vi "Actor Core.vi"(8 "error in":errorcluster, 11 "UserInterface in":refnum<class "UserInterface.lvclass">) -> (0 "error out":errorcluster, 3 "Actor out":refnum<class "Actor.lvclass">)   [LabVIEW 2022 SP3, in "UserInterface.lvlib" / "UserInterface.lvclass"]
doc: "(<B>Filename</B>: Actor Framework.lvlib:Actor.lvclass:Actor Core.vi)\n\nReceives messages to the actor, reacts to them, and initiates any error handling that may shut the actor down.\n\nDescendant classes may override this VI to append parallel tasks for the actor to complete while it handles messages. Overrides use the Call Parent Class Method node."
uses:
  UserInterface.lvclass
  C:/Program Files/National Instruments/LabVIEW 2022/vi.lib/ActorFramework/Actor/Actor.lvclass
  <vilib>/ActorFramework/Actor/Actor.lvclass
  Typedefs/Image Formats.ctl
  Helper Loop Status.ctl
  UserInterface.lvclass/UserInterface.ctl
  <vilib>/ActorFramework/Actor/Actor.lvclass/Actor.ctl
  UI - Controller -- Interface Messages/Component Name Msg/Component Name Msg.lvclass/Component Name Msg.ctl
  <vilib>/ActorFramework/Message Enqueuer/Message Enqueuer.lvclass/Message Enqueuer.ctl
  UI - Controller -- Interface Messages/Total Images Msg/Total Images Msg.lvclass/Total Images Msg.ctl
  UI - Controller -- Interface Messages/Image Type Msg/Image Type Msg.lvclass/Image Type Msg.ctl
  UserInterface Messages/Total Images Msg/Total Images Msg.lvclass/Total Images Msg.ctl
  UI - Controller -- Interface Messages/Image Indicator Ref Msg/Image Indicator Ref Msg.lvclass/Image Indicator Ref Msg.ctl
  UI - Controller -- Interface Messages/Display Image Msg/Display Image Msg.lvclass/Display Image Msg.ctl
  <vilib>/ActorFramework/Message Enqueuer/Enqueue.vi
  <vilib>/ActorFramework/Message Enqueuer/Init from Existing Queue.vi
  UI - Controller -- Interface Messages/Component Name Msg/Component Name Msg.lvclass
  C:/Program Files/National Instruments/LabVIEW 2022/vi.lib/ActorFramework/Message/Message.lvclass
  UI - Controller -- Interface Messages/Total Images Msg/Total Images Msg.lvclass
  UI - Controller -- Interface Messages/Image Type Msg/Image Type Msg.lvclass
  UI - Controller -- Interface Messages/StartHarvest Msg/StartHarvest Msg.lvclass
  UI - Controller -- Interface Messages/StopHarvest Msg/StopHarvest Msg.lvclass
  UserInterface Messages/Total Images Msg/Total Images Msg.lvclass
  UI - Controller -- Interface Messages/Launch Calibration Msg/Launch Calibration Msg.lvclass
  UI - Controller -- Interface Messages/Image Request Msg/Image Request Msg.lvclass
  UI - Controller -- Interface Messages/Launch Settings Msg/Launch Settings Msg.lvclass
  UI - Controller -- Interface Messages/Open Folder Msg/Open Folder Msg.lvclass
  UI - Controller -- Interface Messages/Image Indicator Ref Msg/Image Indicator Ref Msg.lvclass
  UserInterface Messages/Reset UI Msg/Reset UI Msg.lvclass
  <vilib>/ActorFramework/Stop Msg/Stop Msg.lvclass
  UI - Controller -- Interface Messages/Display Image Msg/Display Image Msg.lvclass
  <vilib>/ActorFramework/Message Priority Queue/Priority Enqueue.vi
  <vilib>/ActorFramework/Message Enqueuer/Message Enqueuer.lvclass
  UserInterface.lvlib
panel:
  out "PLC":bool caption="PLC Not Ready"
  out "Image Sensor":bool caption="Sensor Not Ready"
  out "Version":string
  in  "Total Images":u32
  in  "Image Format":T1
  in  "Component Name":string
  in  "Open Folder":bool
  in  "Calibration":bool
  in  "Settings":bool
  in  "Stop":bool
  in  "Start":bool
  out "?":string
  in  "Trigger":bool
  in  "Progress":string
  out "Selected Image":T2(plugin-control)
  out "ProgressBar":u32(slide) caption="Click on Start to Acquire Images..." scale=0.0..100.0
  in  "Image List":i32(listbox)
  out "Log":string
  # "Aayvu CT"
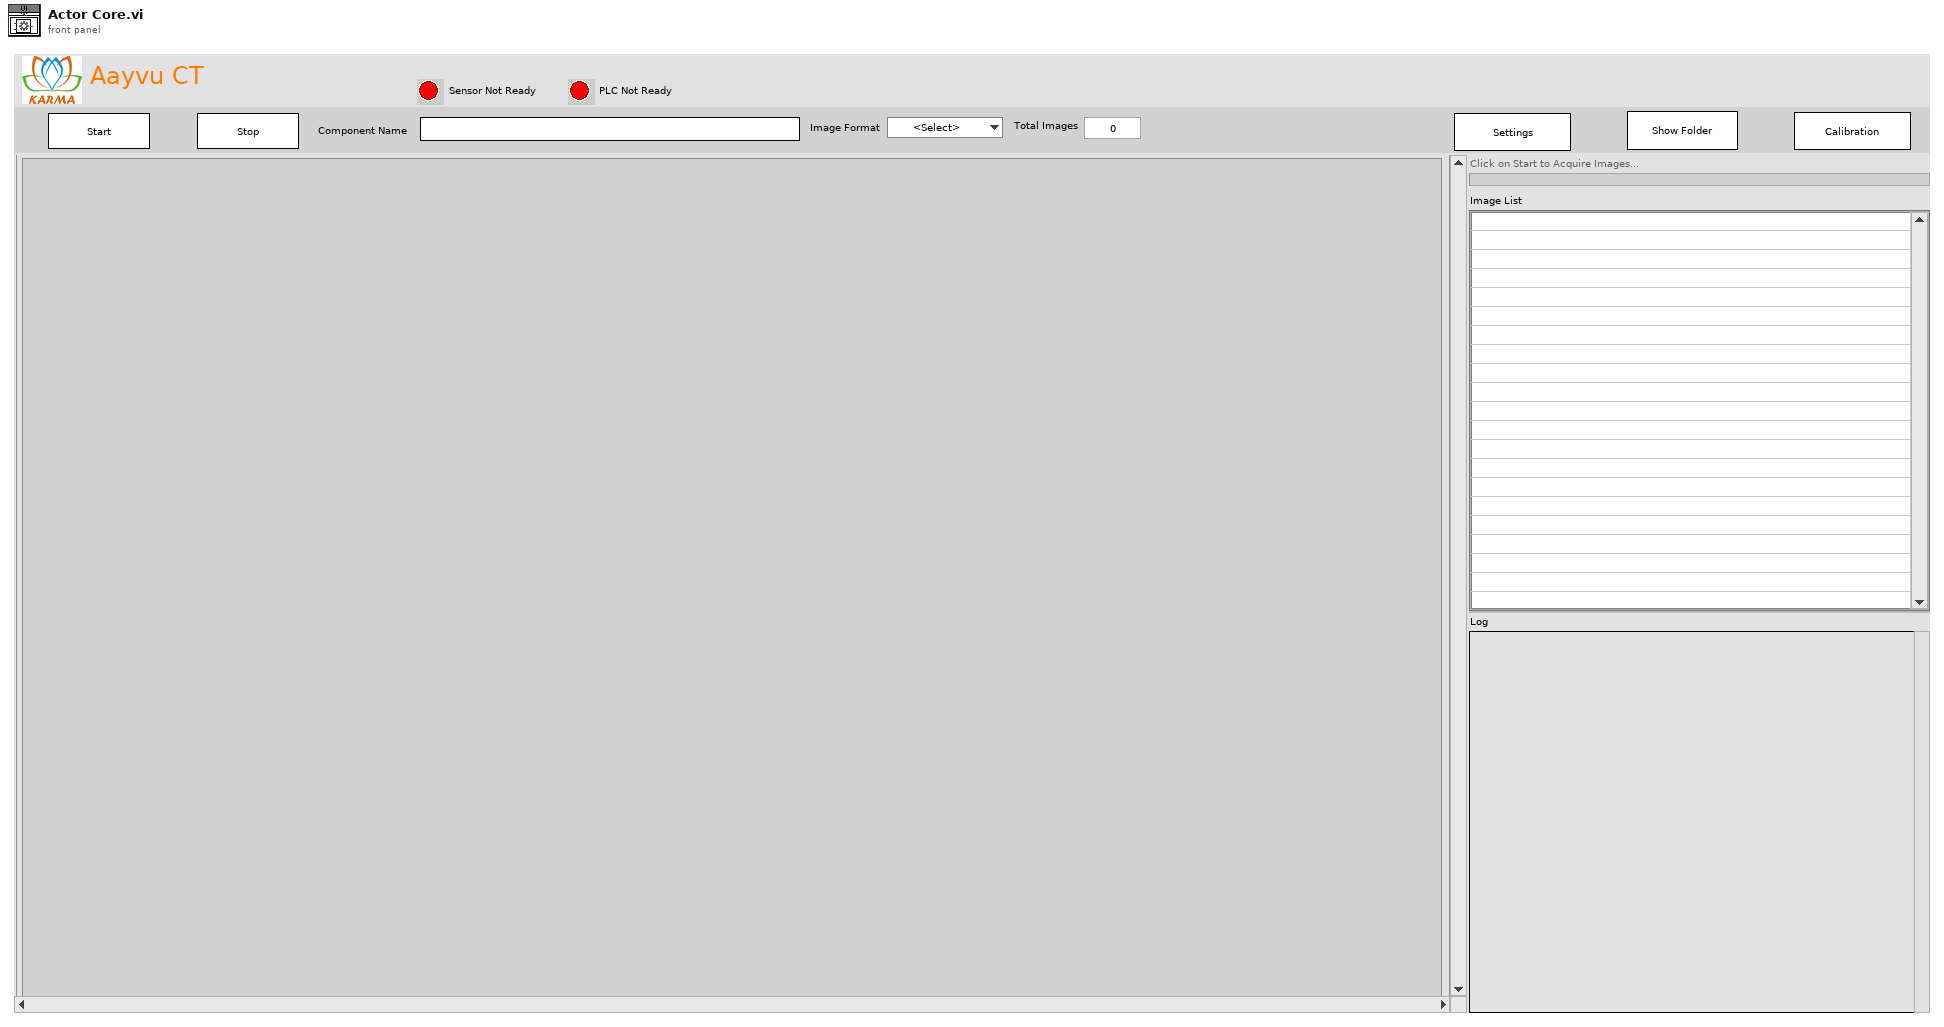
[diagram p1: front panel]
types:
  T1 = typedef "Image Formats.ctl" = enum16{"<Select>", "TIFF", "RAW"}
  T2 = typedef "IMAQ Image.ctl" = refnum<image>
  T3 = enum32{"Invalid", "Standard", "Closed", "Hidden", "Minimized", "Maximized"}
  T4 = cluster{"Image List":refnum<vi>, "ProgressBar":refnum<vi>, "Log":refnum<vi>, "Image Indicator":refnum<vi>}
  T5 = typedef "UserInterface.lvlib/Helper Loop Status.ctl" = enum16{"Poll", "Init", "Update Controls", "Control Status - Start", "Control Status - Stop", "Error", "Exit"}
  T6 = cluster{"Sensor Status":refnum<user-event>, "PLC Status":refnum<user-event>, "ACQ Complete":refnum<user-event>}
  T7 = enum8{"Enabled", "Disabled", "Disabled and Grayed Out"}
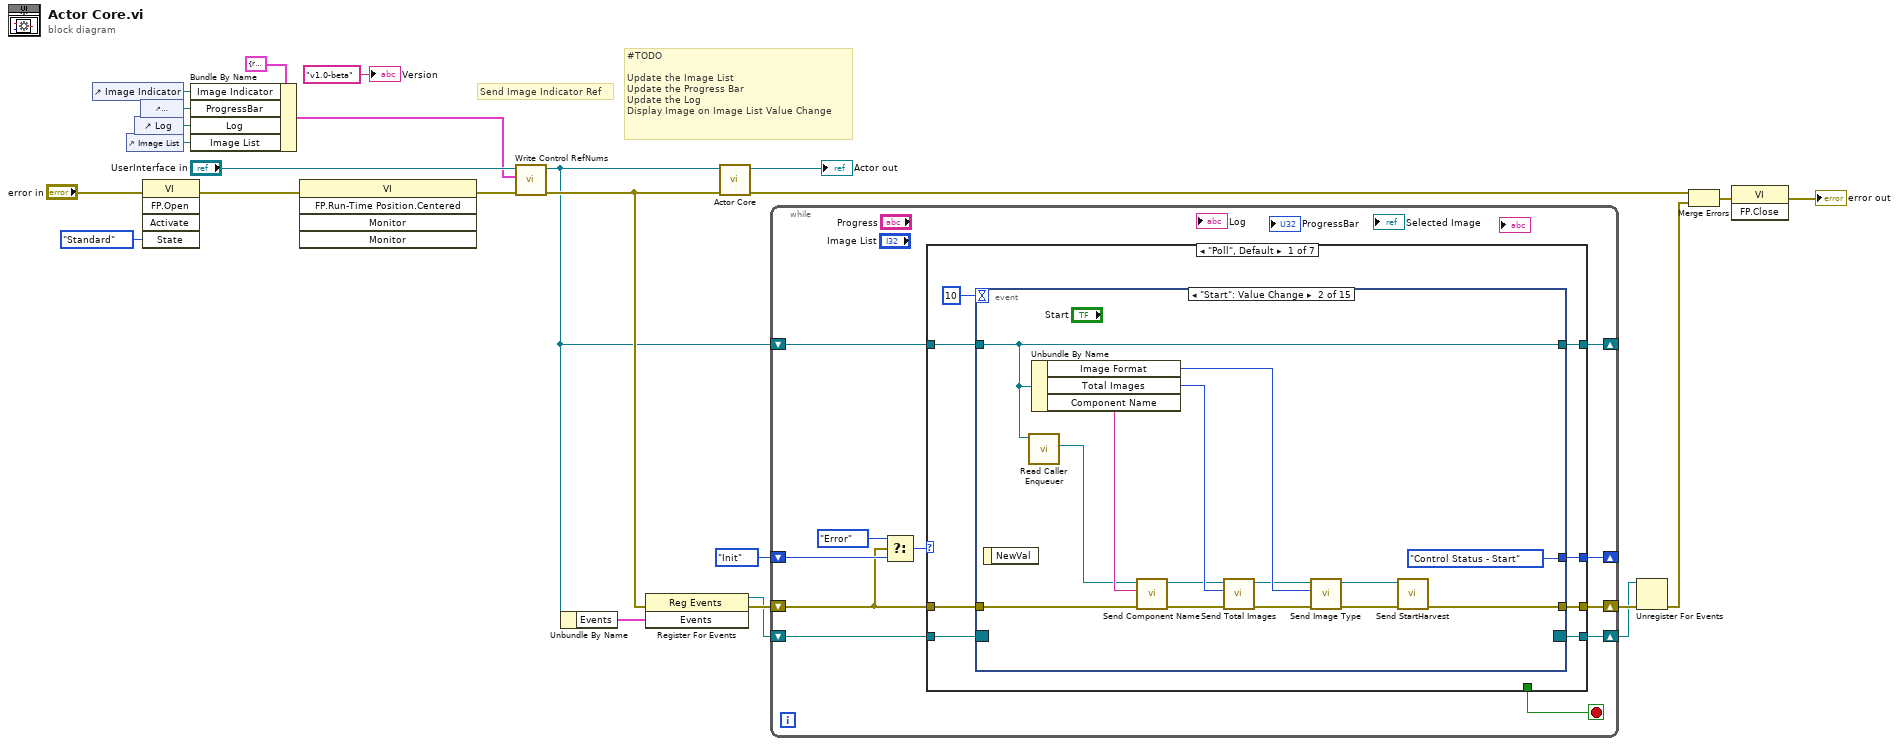
[diagram p0: block diagram]
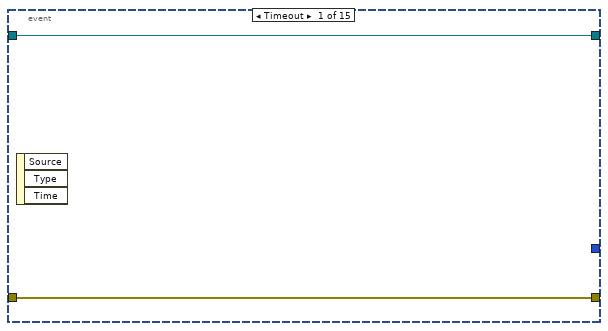
[diagram p2: hidden frame]
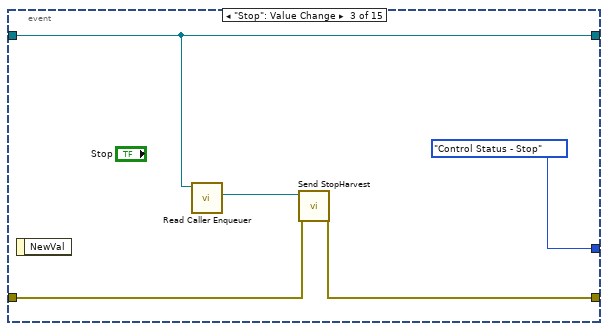
[diagram p3: hidden frame]
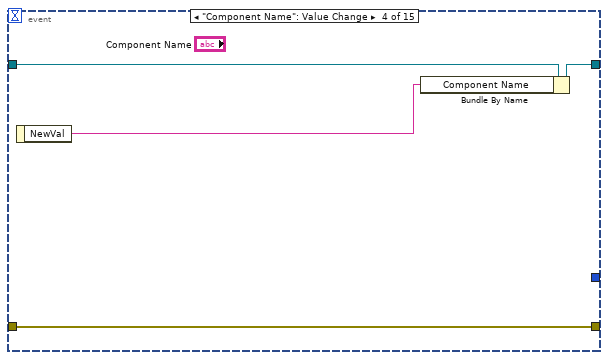
[diagram p4: hidden frame]
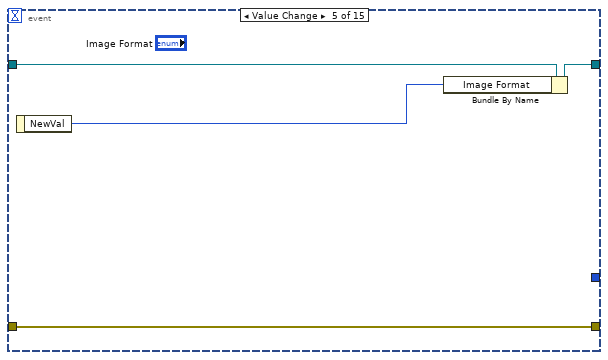
[diagram p5: hidden frame]
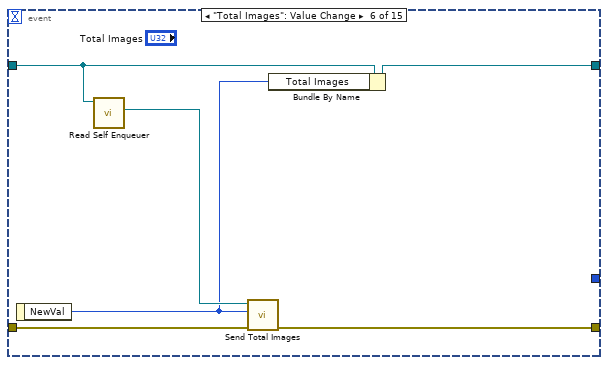
[diagram p6: hidden frame]
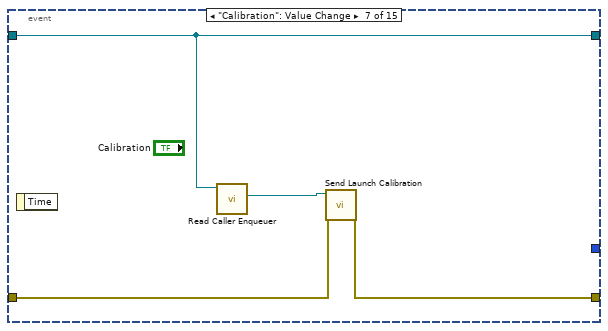
[diagram p7: hidden frame]
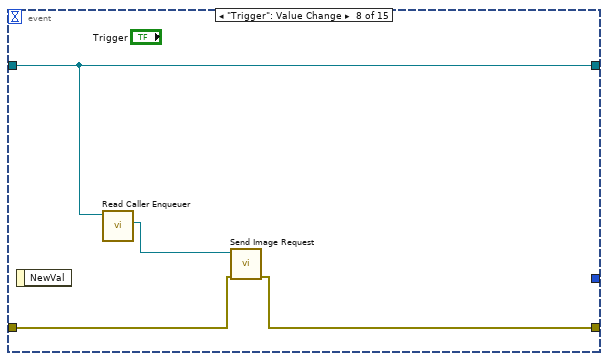
[diagram p8: hidden frame]
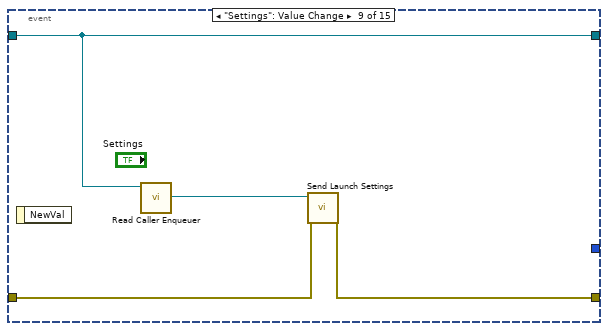
[diagram p9: hidden frame]
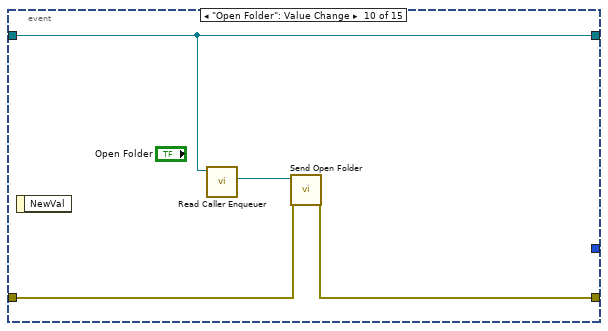
[diagram p10: hidden frame]
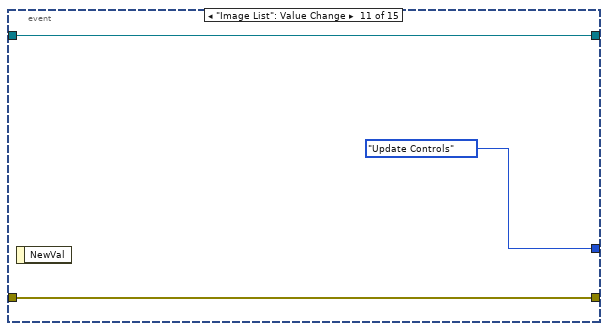
[diagram p11: hidden frame]
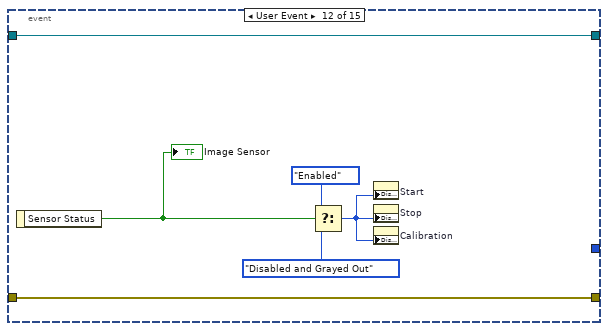
[diagram p12: hidden frame]
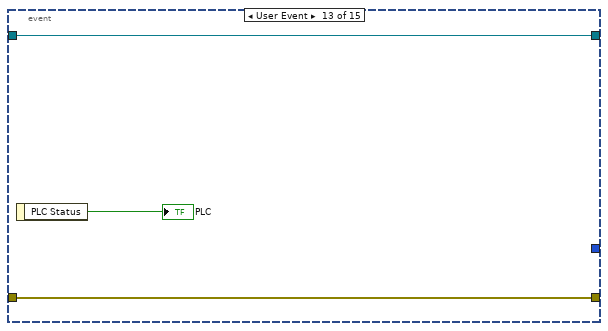
[diagram p13: hidden frame]
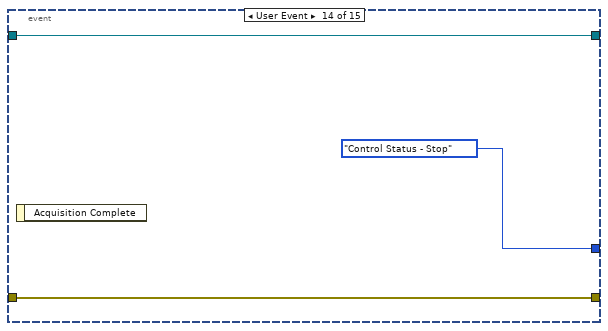
[diagram p14: hidden frame]
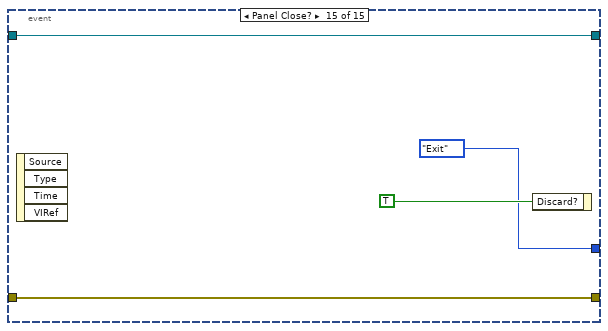
[diagram p15: hidden frame]
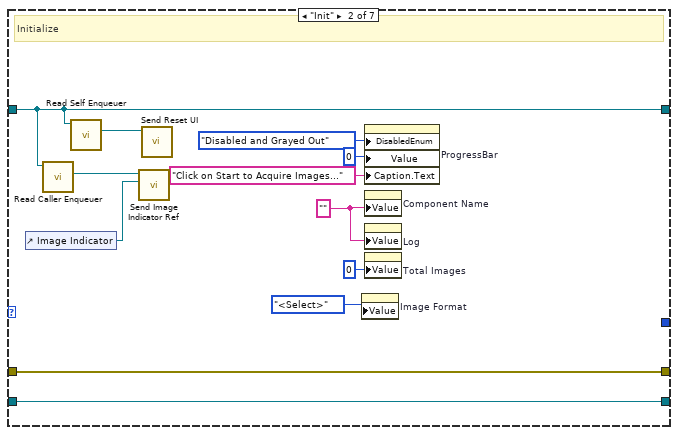
[diagram p16: hidden frame]
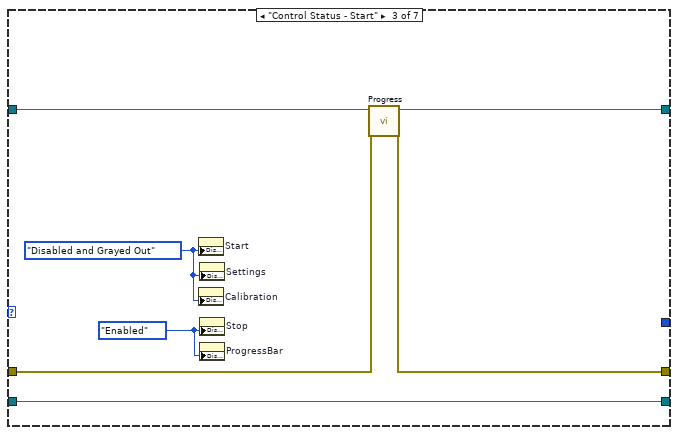
[diagram p17: hidden frame]
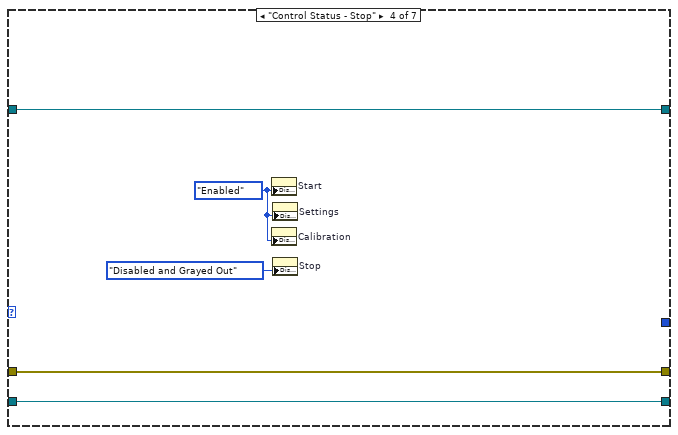
[diagram p18: hidden frame]
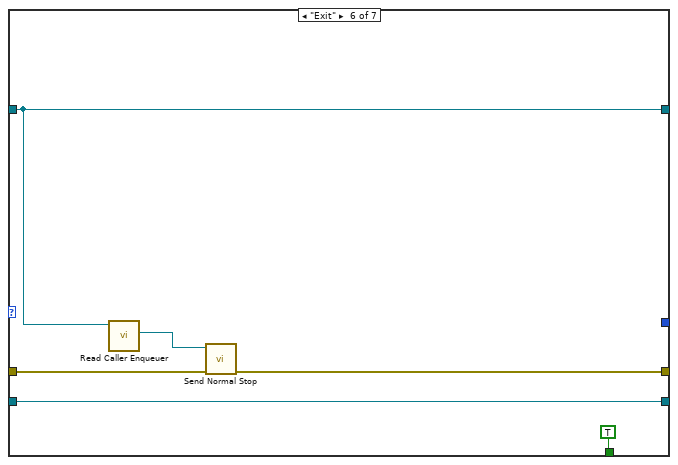
[diagram p20: hidden frame]
diagram:
  # "Send Image Indicator Ref"
  # "#TODO \n\nUpdate the Image List\nUpdate the Progress Bar\nUpdate the Log\nDisplay Image on Image List Value Change"
  n1 = control-ref of="Image Indicator"() -> (w18:refnum<vi>)
  n2 = control-ref of="Image List"() -> (w15:refnum<vi>)
  n3 = control-ref of="Log"() -> (w16:refnum<vi>)
  n4 = control-ref of="ProgressBar"() -> (w17:refnum<vi>)
  n5 = invoke class="VI" method="FP.Open"(error in="error in", "State"=T3."Standard") -> (error out=w4:errorcluster)  [unwired: 3 in, 4 out]
  n6 = Bundle By Name(cluster=T4 {"Image List"=refnum, "ProgressBar"=refnum, "Log"=refnum, "Image Indicator"=refnum} ("Control RefNums"), "Image Indicator"=w18, "ProgressBar"=w17, "Log"=w16, "Image List"=w15) -> (w19:T4)
  n7 = invoke class="VI" method="FP.Run-Time Position.Centered"(error in=w4) -> (error out=w1:errorcluster)  [unwired: 4 in, 4 out]
  n8 = call "Write Control RefNums.vi"("error in (no error)"=w1, "Control RefNums"=w19, "UserInterface in"="UserInterface in") -> ("error out"=w14:errorcluster, "UserInterface out"=w9:refnum<class "UserInterface.lvclass">)  [unwired: 7 in]
  n9 = Unbundle By Name(w9) -> ("Events"=w8:T6)
  n10 = register-events(error in=w14, w8) -> (reference out=w12:refnum<event-registration>, error out=w13:errorcluster)  [unwired: 1 in]
  n11 = call-parent "Actor Core.vi"("error in"=w14, "Actor in"=w9) -> ("error out"=w7:errorcluster, "Actor out"=→"Actor out":refnum<class "Actor.lvclass">)  [unwired: 8 in]
  n12 = while {
    shift-right: [w36] -> _
    shift-left: Helper_Loop_Status."Init" -> [w32]
    shift-right: [w33] -> _
    shift-left: w9 -> [w35]
    shift-right: [w29] -> w11
    shift-left: w13 -> [w30]
    shift-right: [w27] -> w10
    shift-left: w12 -> [w28]
    stop <- w34 stop-if-true
    n13 = Select(t=Helper_Loop_Status."Error", s=w30, f=w32) -> (s? t:f=w31:T5)
    n14 = case shown="\"Poll\", Default" w31 {
      tunnel: [w44 _ _ _ _ _ _] -> w36
      tunnel: w35 -> [w42 w119 w131 w138 w141 w145 w152]
      tunnel: [_ _ _ _ _ TRUE _] -> w34
      tunnel: [w41 w119 w130 w138 w141 w145 w152] -> w33
      tunnel: w30 -> [w40 w126 w129 w137 w140 w143 w157]
      tunnel: [w39 w126 w128 w137 w140 w142 w149] -> w29
      tunnel: w28 -> [w38 w125 w133 w136 w139 w146 w156]
      tunnel: [w37 w125 w133 w136 w139 w146 w156] -> w27
      frame "Poll", Default {
        n15 = event shown="[1] \"Start\": Value Change" {
          selector: w38 -> [_ _ _ _ _ _ _ _ _ _ _ _ _ _ _]
          dyn-events: [_ _ _ _ _ _ _ _ _ _ _ _ _ _ _] -> w37
          timeout: 10 -> [_ _ _ _ _ _ _ _ _ _ _ _ _ _ _]
          tunnel: [_ Helper_Loop_Status."Control Status - Start" Helper_Loop_Status."Control Status - Stop" _ _ _ _ _ _ _ Helper_Loop_Status."Update Controls" _ _ Helper_Loop_Status."Control Status - Stop" Helper_Loop_Status."Exit"] -> w44
          tunnel: w42 -> [w46 w58 w65 w69 w73 w78 w83 w87 w91 w95 w98 w104 w107 w110 w113]
          tunnel: [w46 w58 w65 w67 w71 w79 w83 w87 w91 w95 w98 w104 w107 w110 w113] -> w41
          tunnel: w40 -> [w45 w53 w63 w68 w72 w75 w81 w85 w89 w93 w97 w103 w106 w109 w112]
          tunnel: [w45 w60 w62 w68 w72 w74 w80 w84 w88 w92 w97 w103 w106 w109 w112] -> w39
          event Timeout {
            n16 = event-data() -> ()  [unwired: 1 in, 3 out]
          }
          event "Start": Value Change {
            n17 = event-data() -> ()  [unwired: 1 in, 1 out]
            n18 = call <vilib>:"Read Caller Enqueuer.vi"("Actor"=w58) -> ("Caller Enqueuer"=w55:refnum<class "Message Enqueuer.lvclass">)  [unwired: 10 in]
            n19 = Unbundle By Name(w58) -> ("Image Format"=w54:T1, "Total Images"=w57:u32, "Component Name"=w56:string)
            n20 = call "Send Component Name.vi"("error in (no error)"=w53, "Component Name"=w56, "Message Enqueuer"=w55) -> ("error out"=w52:errorcluster, "Message Enqueuer out"=w50:refnum<class "Message Enqueuer.lvclass">)  [unwired: 7 in]
            n21 = call "Send Total Images.vi"("error in (no error)"=w52, "Total Images"=w57, "Message Enqueuer"=w50) -> ("error out"=w51:errorcluster, "Message Enqueuer out"=w49:refnum<class "Message Enqueuer.lvclass">)  [unwired: 7 in]
            n22 = call "Send Image Type.vi"("error in (no error)"=w51, "Image Type"=w54, "Message Enqueuer"=w49) -> ("error out"=w47:errorcluster, "Message Enqueuer out"=w48:refnum<class "Message Enqueuer.lvclass">)  [unwired: 7 in]
            n23 = call "Send StartHarvest.vi"("error in (no error)"=w47, "Message Enqueuer"=w48) -> ("error out"=w60:errorcluster)  [unwired: 8 in, 1 out]
          }
          event "Stop": Value Change {
            n24 = event-data() -> ()  [unwired: 1 in, 1 out]
            n25 = call <vilib>:"Read Caller Enqueuer.vi"("Actor"=w65) -> ("Caller Enqueuer"=w64:refnum<class "Message Enqueuer.lvclass">)  [unwired: 10 in]
            n26 = call "Send StopHarvest.vi"("error in (no error)"=w63, "Message Enqueuer"=w64) -> ("error out"=w62:errorcluster)  [unwired: 8 in, 1 out]
          }
          event "Component Name": Value Change {
            n27 = event-data() -> ("NewVal"=w66:string)  [unwired: 1 in]
            n28 = Bundle By Name(cluster=w69, "Component Name"=w66) -> (w67:refnum<class "UserInterface.lvclass">)
          }
          event Value Change {
            n29 = event-data() -> ("NewVal"=w70:T1)  [unwired: 1 in]
            n30 = Bundle By Name(cluster=w73, "Image Format"=w70) -> (w71:refnum<class "UserInterface.lvclass">)
          }
          event "Total Images": Value Change {
            n31 = event-data() -> ("NewVal"=w76:u32)  [unwired: 1 in]
            n32 = call <vilib>:"Read Self Enqueuer.vi"("Actor"=w78) -> ("Self Enqueuer"=w77:refnum<class "Message Enqueuer.lvclass">)  [unwired: 10 in]
            n33 = call "Send Total Images.vi"("error in (no error)"=w75, "Total Images"=w76, "Message Enqueuer"=w77) -> ("error out"=w74:errorcluster)  [unwired: 7 in, 1 out]
            n34 = Bundle By Name(cluster=w78, "Total Images"=w76) -> (w79:refnum<class "UserInterface.lvclass">)
          }
          event "Calibration": Value Change {
            n35 = event-data() -> ()  [unwired: 1 in, 1 out]
            n36 = call <vilib>:"Read Caller Enqueuer.vi"("Actor"=w83) -> ("Caller Enqueuer"=w82:refnum<class "Message Enqueuer.lvclass">)  [unwired: 10 in]
            n37 = call "Send Launch Calibration.vi"("error in (no error)"=w81, "Message Enqueuer"=w82) -> ("error out"=w80:errorcluster)  [unwired: 8 in, 1 out]
          }
          event "Trigger": Value Change {
            n38 = event-data() -> ()  [unwired: 1 in, 1 out]
            n39 = call <vilib>:"Read Caller Enqueuer.vi"("Actor"=w87) -> ("Caller Enqueuer"=w86:refnum<class "Message Enqueuer.lvclass">)  [unwired: 10 in]
            n40 = call "Send Image Request.vi"("error in (no error)"=w85, "Message Enqueuer"=w86) -> ("error out"=w84:errorcluster)  [unwired: 8 in, 1 out]
          }
          event "Settings": Value Change {
            n41 = event-data() -> ()  [unwired: 1 in, 1 out]
            n42 = call <vilib>:"Read Caller Enqueuer.vi"("Actor"=w91) -> ("Caller Enqueuer"=w90:refnum<class "Message Enqueuer.lvclass">)  [unwired: 10 in]
            n43 = call "Send Launch Settings.vi"("error in (no error)"=w89, "Message Enqueuer"=w90) -> ("error out"=w88:errorcluster)  [unwired: 8 in, 1 out]
          }
          event "Open Folder": Value Change {
            n44 = event-data() -> ()  [unwired: 1 in, 1 out]
            n45 = call <vilib>:"Read Caller Enqueuer.vi"("Actor"=w95) -> ("Caller Enqueuer"=w94:refnum<class "Message Enqueuer.lvclass">)  [unwired: 10 in]
            n46 = call "Send Open Folder.vi"("error in (no error)"=w93, "Message Enqueuer"=w94) -> ("error out"=w92:errorcluster)  [unwired: 8 in, 1 out]
          }
          event "Image List": Value Change {
            n47 = event-data() -> ()  [unwired: 1 in, 1 out]
          }
          event User Event {
            n48 = event-data() -> ("Sensor Status"=w102:bool)  [unwired: 1 in]
            "Image Sensor" <- w102
            n49 = Select(t=T7."Enabled" ("Disabled"), s=w102, f=T7."Disabled and Grayed Out" ("Disabled")) -> (s? t:f=w99:T7)
            n50 = property on="Start" class="Bool"("DisabledEnum"=w99) -> ()  [unwired: 2 in, 2 out]
            n51 = property on="Stop" class="Bool"("DisabledEnum"=w99) -> ()  [unwired: 2 in, 2 out]
            n52 = property on="Calibration" class="Bool"("DisabledEnum"=w99) -> ()  [unwired: 2 in, 2 out]
          }
          event User Event {
            n53 = event-data() -> ("PLC Status"=→"PLC":bool)  [unwired: 1 in]
          }
          event User Event {
            n54 = event-data() -> ()  [unwired: 1 in, 1 out]
          }
          event Panel Close? {
            n55 = event-data() -> ()  [unwired: 1 in, 4 out]
            n56 = event-data("Discard?"=TRUE) -> ()  [unwired: 1 in, 1 out]
          }
        }
      }
      frame "Init" {
        w117 = "" ("Log")
        # "Initialize"
        n57 = control-ref of="Image Indicator"() -> (w120:refnum<vi>)
        n58 = call <vilib>:"Read Caller Enqueuer.vi"("Actor"=w119) -> ("Caller Enqueuer"=w121:refnum<class "Message Enqueuer.lvclass">)  [unwired: 10 in]
        n59 = call <vilib>:"Read Self Enqueuer.vi"("Actor"=w119) -> ("Self Enqueuer"=w118:refnum<class "Message Enqueuer.lvclass">)  [unwired: 10 in]
        n60 = call "Send Image Indicator Ref.vi"("Ctl Refnum"=w120, "Message Enqueuer"=w121) -> ()  [unwired: 8 in, 2 out]
        n61 = call "Send Reset UI.vi"("Message Enqueuer"=w118) -> ()  [unwired: 9 in, 2 out]
        n62 = property on="Image Format" class="Enum (strict)"("Value"=Image_Formats."<Select>" ("Image Format")) -> ()  [unwired: 2 in, 2 out]
        n63 = property on="ProgressBar" class="Slide (strict)"("DisabledEnum"=T7."Disabled and Grayed Out" ("Disabled"), "Value"=u32 0 ("ProgressBar"), "Caption.Text"="Click on Start to Acquire Images...") -> ()  [unwired: 2 in, 2 out]
        n64 = property on="Component Name" class="Str"("Value"=w117) -> ()  [unwired: 2 in, 2 out]
        n65 = property on="Log" class="Str"("Value"=w117) -> ()  [unwired: 2 in, 2 out]
        n66 = property on="Total Images" class="DigNum (strict)"("Value"=u32 0 ("Total Images")) -> ()  [unwired: 2 in, 2 out]
      }
      frame "Control Status - Start" {
        w127 = T7."Enabled" ("Disabled")
        w132 = T7."Disabled and Grayed Out" ("Disabled")
        n67 = property on="Start" class="Bool"("DisabledEnum"=w132) -> ()  [unwired: 2 in, 2 out]
        n68 = property on="Calibration" class="Bool"("DisabledEnum"=w132) -> ()  [unwired: 2 in, 2 out]
        n69 = property on="Settings" class="Bool"("DisabledEnum"=w132) -> ()  [unwired: 2 in, 2 out]
        n70 = property on="Stop" class="Bool"("DisabledEnum"=w127) -> ()  [unwired: 2 in, 2 out]
        n71 = property on="ProgressBar" class="Slide (strict)"("DisabledEnum"=w127) -> ()  [unwired: 2 in, 2 out]
        n72 = call "Progress.vi"("error in"=w129, "UserInterface in"=w131) -> ("error out"=w128:errorcluster, "UserInterface out"=w130:refnum<class "UserInterface.lvclass">)  [unwired: 8 in]
      }
      frame "Control Status - Stop" {
        w135 = T7."Enabled" ("Disabled")
        n73 = property on="Start" class="Bool"("DisabledEnum"=w135) -> ()  [unwired: 2 in, 2 out]
        n74 = property on="Calibration" class="Bool"("DisabledEnum"=w135) -> ()  [unwired: 2 in, 2 out]
        n75 = property on="Settings" class="Bool"("DisabledEnum"=w135) -> ()  [unwired: 2 in, 2 out]
        n76 = property on="Stop" class="Bool"("DisabledEnum"=T7."Disabled and Grayed Out" ("Disabled")) -> ()  [unwired: 2 in, 2 out]
      }
      frame "Error" {
      }
      frame "Exit" {
        n77 = call <vilib>:"Read Caller Enqueuer.vi"("Actor"=w145) -> ("Caller Enqueuer"=w144:refnum<class "Message Enqueuer.lvclass">)  [unwired: 10 in]
        n78 = call <vilib>:"Send Normal Stop.vi"("error in (no error)"=w143, "Message Enqueuer"=w144) -> ("error out"=w142:errorcluster)  [unwired: 9 in]
      }
      frame "Update Controls" {
        n79 = Unbundle By Name(w152) -> ("Image List"=w155:refnum<vi>)
        n80 = call <vilib>:"Read Caller Enqueuer.vi"("Actor"=w152) -> ("Caller Enqueuer"=w151:refnum<class "Message Enqueuer.lvclass">)  [unwired: 10 in]
        n81 = property class="LstBox (strict)"(reference=w155, error in=w157) -> (error out=w150:errorcluster, "Item Names"=w154:string[], "Value"=w153:i32)  [unwired: 1 out]
        n82 = Index Array(array=w154, index=w153) -> (element=w148:string)
        n83 = call "Send Display Image.vi"("error in (no error)"=w150, "File Name"=w148, "Message Enqueuer"=w151) -> ("error out"=w149:errorcluster)  [unwired: 7 in, 1 out]
      }
    }
  }
  n84 = Unregister For Events(event registration refnum=w10, error in=w11) -> (error out=w6:errorcluster)
  n85 = Merge Errors(w7, w6) -> (w5:errorcluster)
  n86 = invoke class="VI" method="FP.Close"(error in=w5) -> (error out=→"error out":errorcluster)  [unwired: 2 in, 2 out]
  "Version" <- "v1.0-beta" ("Version")
